vi "IP Connection Sandbox.vi"() -> ()   [LabVIEW 2011]
uses:
  Classes/IP Connection/Type Definitions/Get Stack ID Response.ctl
  Classes/Device/Type Definitions/Firmware Version.ctl
  Classes/IP Connection/Type Definitions/Enumerate CB.ctl
  Classes/IP Connection/Properties/Read Enumerate Callback.vi
  Classes/IP Connection/IP Connection.lvclass
  Classes/Device/Device.lvclass
panel:
  out "timed out":bool
  out "Sucessful":bool
  out "Devices":T1[](array[typedef])
  out "Get Stack ID Response":T2
  in  "Device UID":string
  in  "Get Stack ID":bool
  out "Device Count":i32
  in  "Enumerate":bool
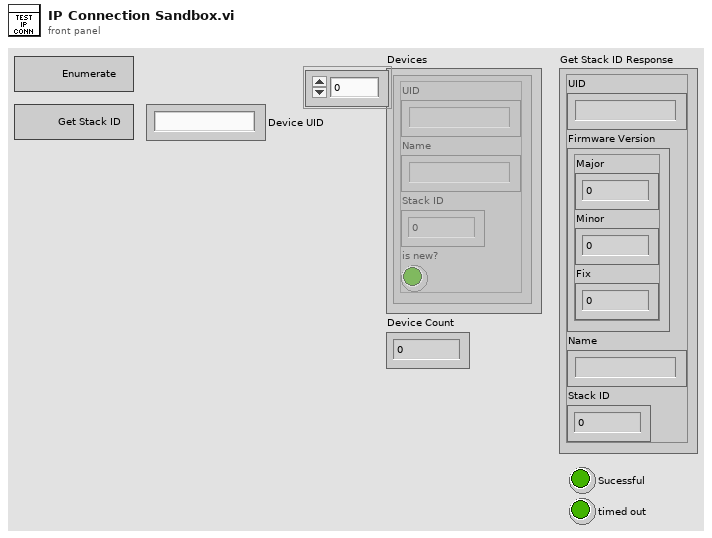
[diagram p1: front panel]
types:
  T1 = typedef "Tinkerforge.lvlib/IP Connection.lvclass/Enumerate CB.ctl" = cluster{"UID":string, "Name":string, "Stack ID":u8, "is new?":bool}
  T2 = typedef "Tinkerforge.lvlib/IP Connection.lvclass/Get Stack ID Response.ctl" = cluster{"UID":string, "Firmware Version":T3, "Name":string, "Stack ID":u8}
  T3 = typedef "Tinkerforge.lvlib/Device.lvclass/Firmware Version.ctl" = cluster{"Major":u8, "Minor":u8, "Fix":u8}
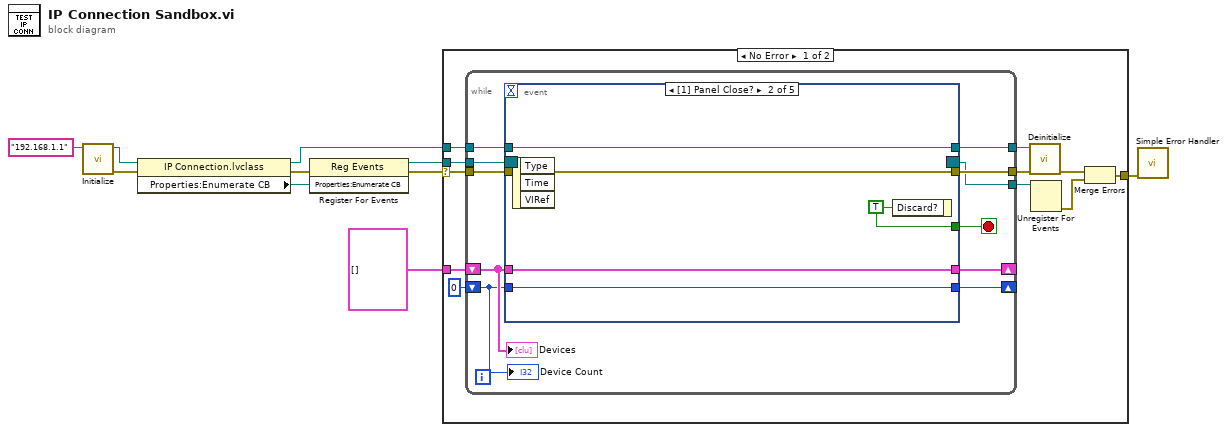
[diagram p0: block diagram]
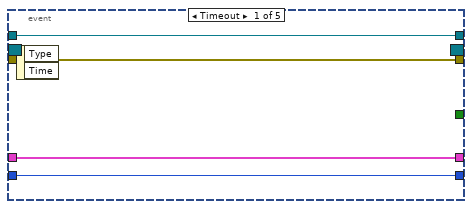
[diagram p2: hidden frame]
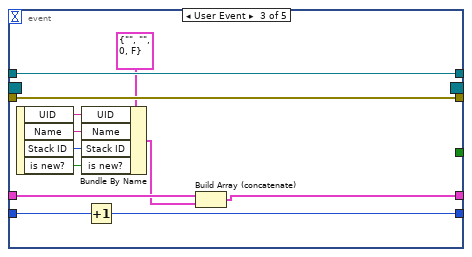
[diagram p3: hidden frame]
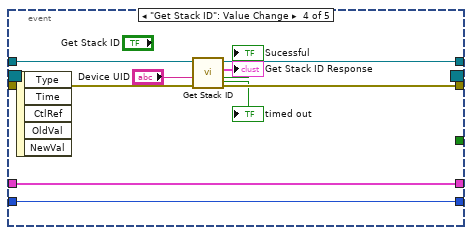
[diagram p4: hidden frame]
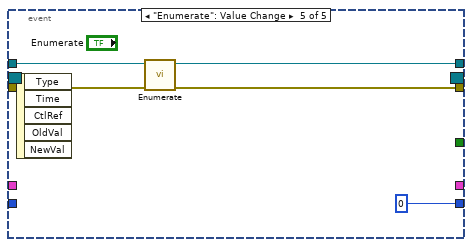
[diagram p5: hidden frame]
diagram:
  n1 = call "Initialize.vi"("IP (localhost)"="192.168.1.1") -> ("error out"=w8:errorcluster, "IP Connection out"=w10:refnum<class "IP Connection.lvclass">)  [unwired: 9 in]
  n2 = property class="IP Connection.lvclass"(reference=w10, error in=w8) -> (reference out=w9:refnum<class "IP Connection.lvclass">, error out=w7:errorcluster, "Properties:Enumerate CB"=w6:refnum<user-event>)
  n3 = register-events(error in=w7, w6) -> (reference out=w5:refnum<event-registration>, error out=w1:errorcluster)  [unwired: 1 in]
  n4 = case shown="No Error" w1 {
    selector: w1 -> [w11 w69]
    tunnel: w9 -> [w19 _]
    tunnel: w5 -> [w18 _]
    tunnel: [w14 w69] -> w4
    tunnel: T1[] [] -> [w12 _]
    frame No Error {
      n5 = while {
        tunnel: w11 -> [w32]
        tunnel: w19 -> [w31]
        tunnel: [w30] -> w21
        tunnel: [w29] -> w20
        tunnel: w18 -> [w28]
        tunnel: [w27] -> w17
        shift-right: [w24] -> _
        shift-left: 0 -> [w23]
        shift-right: [w25] -> _
        shift-left: w12 -> [w26]
        stop <- w22 stop-if-true
        n6 = event shown="[1] Panel Close?" {
          selector: w28 -> [_ _ _ _ _]
          dyn-events: [_ _ _ _ _] -> w27
          timeout: _ -> [_ _ _ _ _]
          tunnel: w32 -> [w35 w40 w52 w61 w68]
          tunnel: w31 -> [w36 w41 w53 w62 w66]
          tunnel: [w36 w41 w53 w59 w65] -> w30
          tunnel: [w35 w40 w52 w60 w67] -> w29
          tunnel: [w34 w39 w50 w63 0] -> w24
          tunnel: w23 -> [w34 w39 w51 w63 _]
          tunnel: w26 -> [w33 w37 w44 w56 _]
          tunnel: [w33 w37 w42 w56 _] -> w25
          tunnel: [_ w38 _ _ _] -> w22
          event Timeout {
            n7 = event-data() -> ()  [unwired: 1 in, 2 out]
          }
          event Panel Close? {
            w38 = TRUE ("Discard?")
            n8 = event-data() -> ()  [unwired: 1 in, 3 out]
            n9 = event-data("Discard?"=w38) -> ()  [unwired: 1 in, 1 out]
          }
          event User Event {
            n10 = event-data() -> ("UID"=w48:string, "Name"=w47:string, "Stack ID"=w46:u8, "is new?"=w45:bool)  [unwired: 1 in]
            n11 = Bundle By Name(cluster=T1 {"UID"="", "Name"="", "Stack ID"=0, "is new?"=FALSE} ("Enumerate CB"), "UID"=w48, "Name"=w47, "Stack ID"=w46, "is new?"=w45) -> (w43:T1)
            n12 = Increment(x=w51) -> (x+1=w50:i32)
            n13 = Build Array (concatenate)(w44, w43) -> (w42:T1[])
          }
          event "Get Stack ID": Value Change {
            n14 = event-data() -> ()  [unwired: 1 in, 5 out]
            n15 = call "Get Stack ID.vi"("error in (no error)"=w61, "Device UID"="Device UID", "IP Connection in"=w62) -> ("error out"=w60:errorcluster, "Sucessful"=→"Sucessful":bool, "Get Stack ID Response"=→"Get Stack ID Response":T2, "IP Connection out"=w59:refnum<class "IP Connection.lvclass">, "timed out"=→"timed out":bool)  [unwired: 4 in]
          }
          event "Enumerate": Value Change {
            n16 = event-data() -> ()  [unwired: 1 in, 5 out]
            n17 = call "Enumerate.vi"("error in (no error)"=w68, "IP Connection in"=w66) -> ("error out"=w67:errorcluster, "IP Connection out"=w65:refnum<class "IP Connection.lvclass">)  [unwired: 8 in]
          }
        }
        "Device Count" <- w23
        "Devices" <- w26
      }
      n18 = call "Deinitialize.vi"("error in (no error)"=w20, "IP Connection in"=w21) -> ("error out"=w16:errorcluster)  [unwired: 9 in]
      n19 = Unregister For Events(event registration refnum=w17) -> (error out=w15:errorcluster)  [unwired: 1 in]
      n20 = Merge Errors(w16, w15) -> (w14:errorcluster)
    }
    frame Error {
    }
  }
  n21 = call <vilib>:"Simple Error Handler.vi"("error in (no error)"=w4) -> ()  [unwired: 4 in, 5 out]
